vi "Init Sub VI.vi"(4 "Device Angle":enum16{"0", "22.5", "45", "67.5", "90"}(ring), 6 "Knob Dia":enum16{"2 in", "3 in", "4 in"}(ring), 7 "Test Type":T2, 8 "String 3":string, 9 "Angle Target":T1, 10 "Magnitude":enum16{"Low", "Medium", "High"}(ring), 11 "Direction":enum16{"CW", "CCW"}(ring)) -> (2 "String":string, 3 "String 2":string)   [LabVIEW 2020]
uses:
  TESTtypedef UPDATED.ctl
  Angle Target NEW type def.ctl
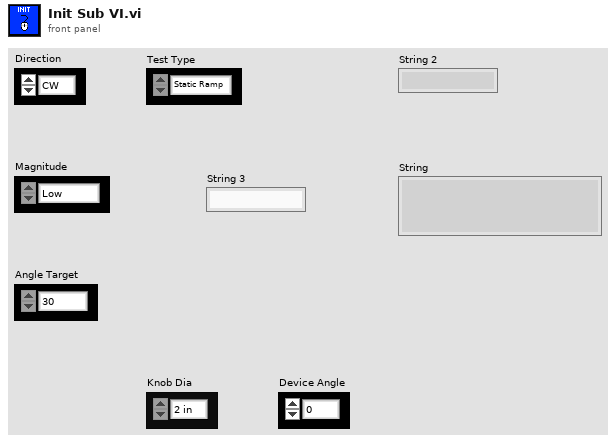
[diagram p1: front panel]
types:
  T1 = typedef "Angle Target NEW type def.ctl" = enum16{"30", "45", "60", "75", "90"}
  T2 = typedef "TESTtypedef UPDATED.ctl" = enum16{"Static Ramp", "Static Sine", "Dynamic"}
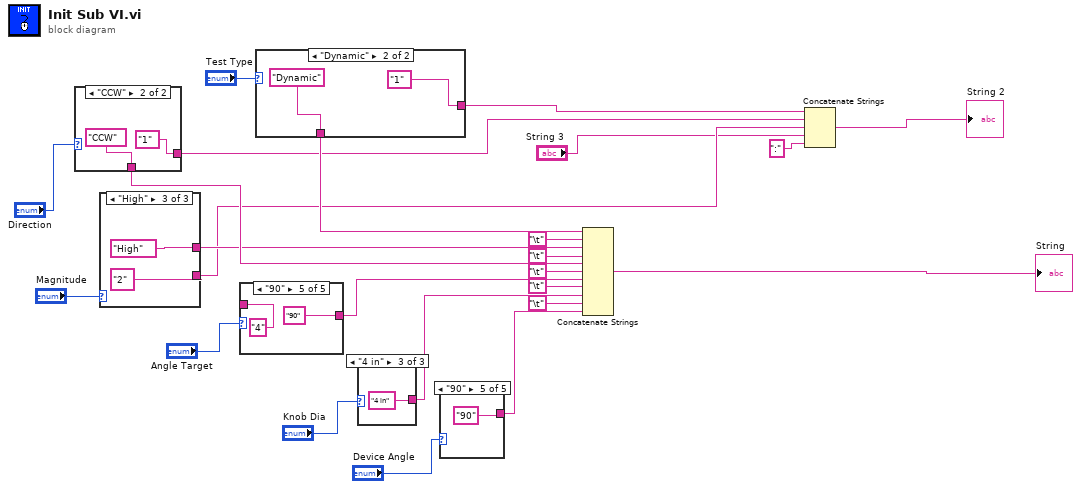
[diagram p0: block diagram]
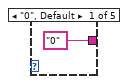
[diagram p2: hidden frame]
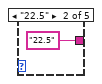
[diagram p3: hidden frame]
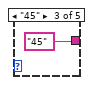
[diagram p4: hidden frame]
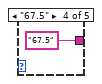
[diagram p5: hidden frame]
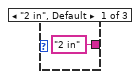
[diagram p6: hidden frame]
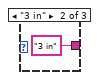
[diagram p7: hidden frame]
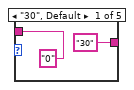
[diagram p8: hidden frame]
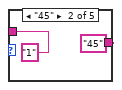
[diagram p9: hidden frame]
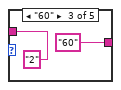
[diagram p10: hidden frame]
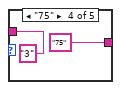
[diagram p11: hidden frame]
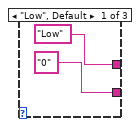
[diagram p12: hidden frame]
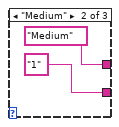
[diagram p13: hidden frame]
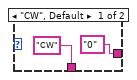
[diagram p14: hidden frame]
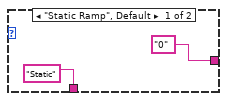
[diagram p15: hidden frame]
diagram:
  n1 = case shown="\"CCW\"" "Direction" {
    tunnel: ["0" "1"] -> w10
    tunnel: ["CW" "CCW"] -> w14
    frame "CW", Default {
    }
    frame "CCW" {
    }
  }
  n2 = case shown="\"High\"" "Magnitude" {
    tunnel: ["0" "1" "2"] -> w4
    tunnel: ["Low" "Medium" "High"] -> w13
    frame "Low", Default {
    }
    frame "Medium" {
    }
    frame "High" {
    }
  }
  n3 = case shown="\"90\"" "Angle Target" {
    tunnel: ["0" "1" "2" "3" "4"] -> _
    tunnel: ["30" "45" "60" "75" "90"] -> w15
    frame "30", Default {
    }
    frame "45" {
    }
    frame "60" {
    }
    frame "75" {
    }
    frame "90" {
    }
  }
  n4 = case shown="\"Dynamic\"" "Test Type" {
    tunnel: ["0" "1"] -> w11
    tunnel: ["Static" "Dynamic"] -> w12
    frame "Static Ramp", Default {
    }
    frame "Dynamic" {
    }
  }
  n5 = case shown="\"4 in\"" "Knob Dia" {
    tunnel: ["2 in" "3 in" "4 in"] -> w17
    frame "2 in", Default {
    }
    frame "3 in" {
    }
    frame "4 in" {
    }
  }
  n6 = case shown="\"90\"" "Device Angle" {
    tunnel: ["0" "22.5" "45" "67.5" "90"] -> w18
    frame "0", Default {
    }
    frame "22.5" {
    }
    frame "45" {
    }
    frame "67.5" {
    }
    frame "90" {
    }
  }
  n7 = Concatenate Strings(w12, "\t", w13, "\t", w14, "\t", w15, "\t", w17, "\t", w18) -> (→"String":string)
  n8 = Concatenate Strings(w11, w10, w4, "String 3", ":" ("string")) -> (→"String 2":string)
